vi "ConvertText.vi"(9 "mode":u8, 11 "Name":string) -> (3 "Array":u8[](array[numeric]) format="%.0x")   [LabVIEW 2016]
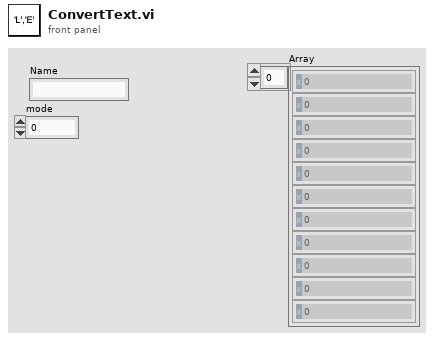
[diagram p1: front panel]
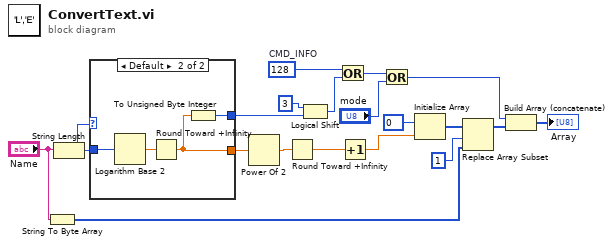
[diagram p0: block diagram]
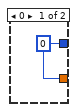
[diagram p2: hidden frame]
diagram:
  w17 = u8 128  # CMD_INFO
  n1 = String To Byte Array(string="Name") -> (unsigned byte array=w10:u8[])
  n2 = String Length(string="Name") -> (length=w3:i32)
  n3 = case shown="Default" w3 {
    tunnel: w3 -> [_ w23]
    tunnel: [w20 w22] -> w4
    tunnel: [w20 w21] -> w2
    frame 0 {
      w20 = u8 0
    }
    frame Default {
      n4 = Logarithm Base 2(1:w23) -> (0:w24:dbl)
      n5 = Round Toward +Infinity(x=w24) -> (ceil(x): smallest int >= x=w21:dbl)
      n6 = To Unsigned Byte Integer(number=w21) -> (unsigned 8bit integer=w22:u8)
    }
  }
  n7 = Power Of 2(x=w2) -> (2^x=w1:dbl)
  n8 = Round Toward +Infinity(x=w1) -> (ceil(x): smallest int >= x=w6:dbl)
  n9 = Logical Shift(y=i16 3, x=w4) -> (x << y=w16:u8)
  n10 = Or(x=w17, y=w16) -> (x .or. y?=w18:u8)
  n11 = Increment(x=w6) -> (x+1=w5:dbl)
  n12 = Or(x=w18, y="mode") -> (x .or. y?=w12:u8)
  n13 = Initialize Array(u8 0 ("CMD_INFO"), w5) -> (w9:u8[])
  n14 = Replace Array Subset(array=w9, new element=w10, index=1) -> (w13:u8[])
  n15 = Build Array (concatenate)(w12, w13) -> (→"Array":u8[])
